vi "buffermgrModule.vi"() -> ()   [LabVIEW 2016]
uses:
  private/vis/BufferStruct.ctl
  private/vis/BUFMGR_actionStruct.ctl
panel:
  in  "error  test 2":errorcluster
  in  "autorelease":string
  in  "maxmem":u64
  in  "error  test":errorcluster
  in  "commandStruct":T1
  in  "send":bool
  in  "local cmds":string="SHUTDOWN"
  out "ConfigFile":path
  in  "log?":bool
  in  "logfile":path=path "/home/arcconfig/MOD_buffmgr.log"
  in  "configvars":string[][](table)=[["BUFF", "minimum", "buffermgrModule.vi", "minbuf", "2", "U16"], ["BUFF", "defsize", "buffermgrModule.vi", "defsize", "1900000", "U64"], ["BUFF", "maxmem", "buffermgrModule.vi", "maxmem", "", "U64"], ["BUFF", "autorelease", "buffermgrModule.vi", "autorelease", "", "STR"], ["LOG", "log", "buffermgrModule.vi", "log?", "no", "BOOL"], ["LOG", "file", "buffermgrModule.vi", "logfile", "", "PATH"]]
  out "error out":errorcluster
  in  "error in":errorcluster
  in  "module name":string="BUFMGR"
  out "automatic buff err":errorcluster
  in  "defsize":u64=19000000 caption="default buffer size"
  in  "minbuf":u16=2 caption="minimum number of free buffres to keep"
  out "stop":bool
  out "Buffers":T2[](array[typedef])
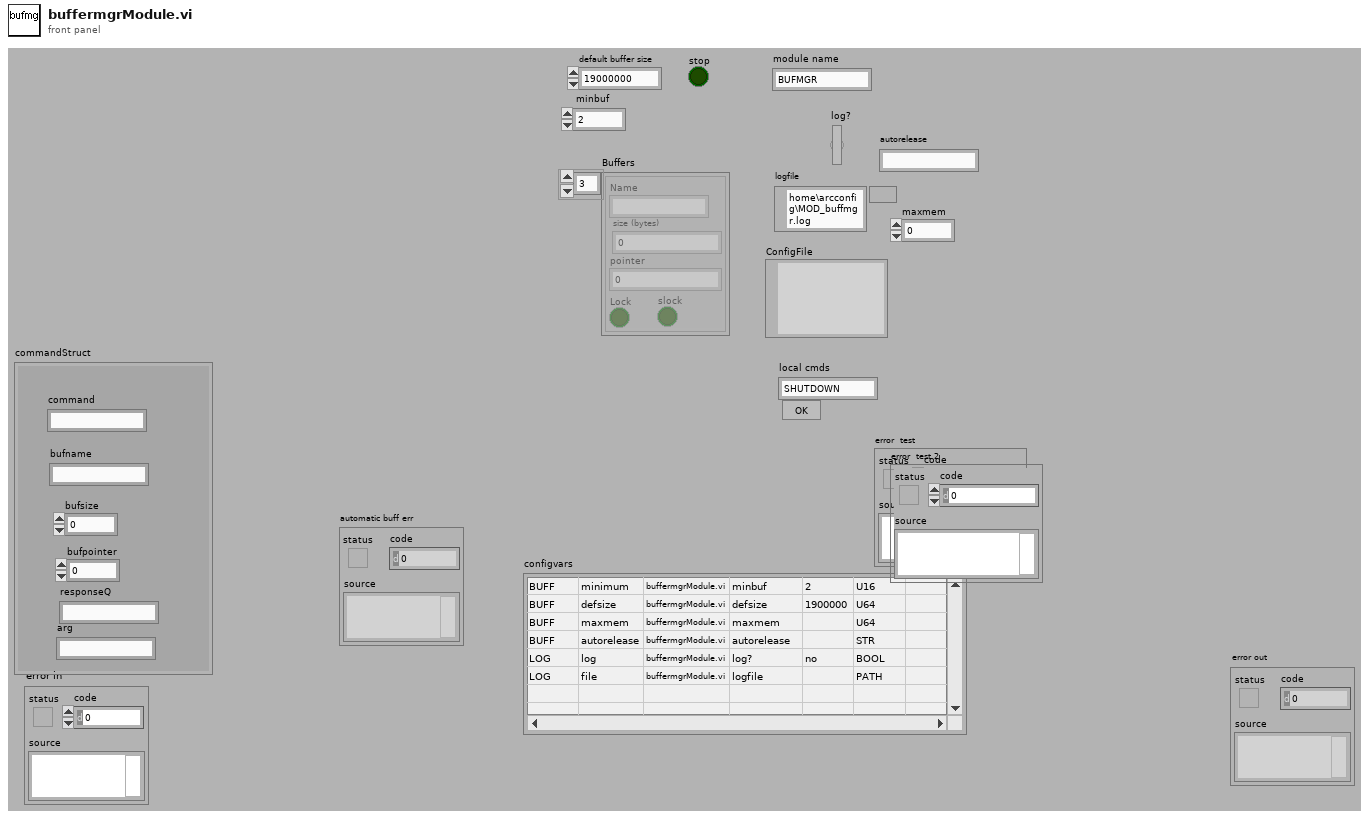
[diagram p1: front panel]
types:
  T1 = cluster{"command":string, "bufname":string, "bufsize":u64, "bufpointer":u64, "responseQ":string, "arg":string}
  T2 = typedef "BufferStruct.ctl" = cluster{"Name":string, "size (bytes)":u64, "pointer":u64, "Lock":bool, "slock":bool}
  T3 = typedef "BUFMGR_actionStruct.ctl" = enum16{"get", "release", "get & lock", "unlock", "release all", "find", "release smaller than", "release bigger than", "release different than", "release equal to", "release unlocked", "info", "get & doublelock", "release secured", "double unlock"}
  T4 = cluster{"pointer":u64, "size":u64, "progress":u32, "status":string}
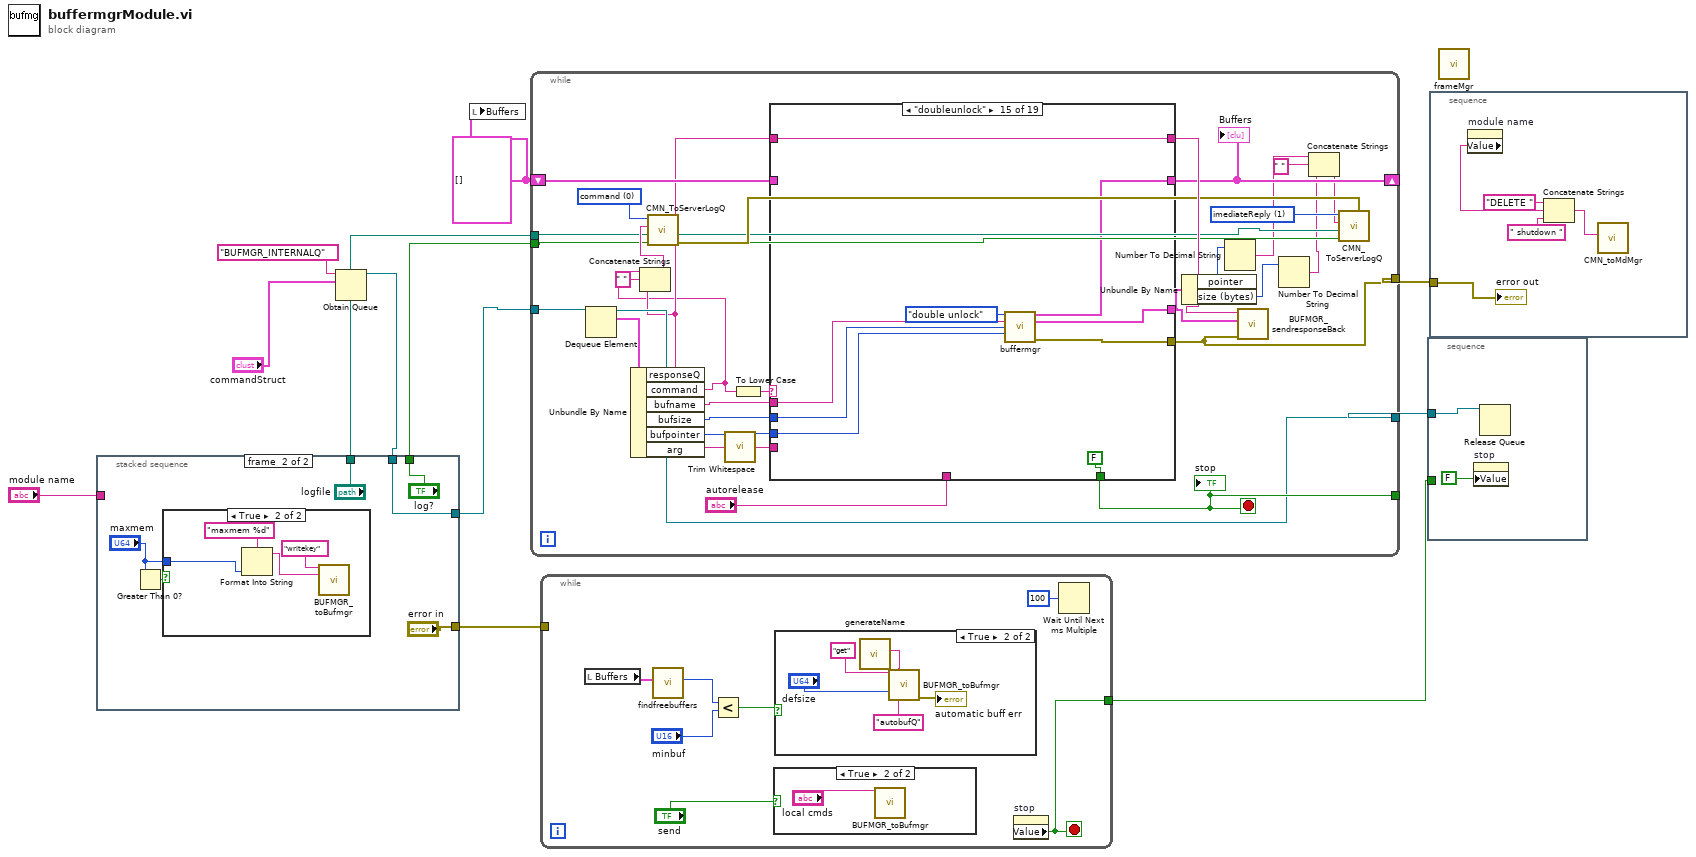
[diagram p0: block diagram]
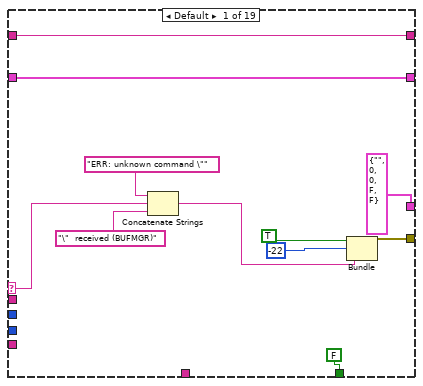
[diagram p2: hidden frame]
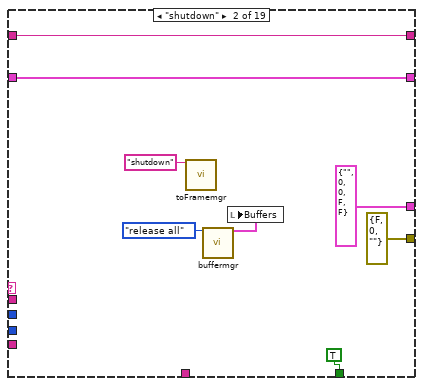
[diagram p3: hidden frame]
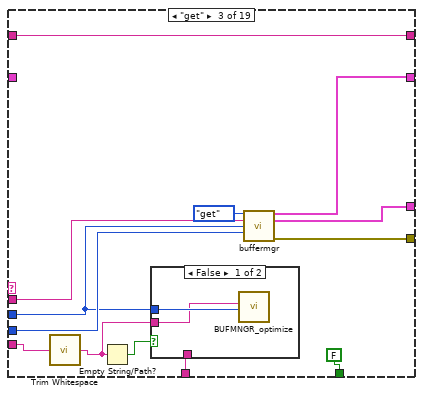
[diagram p4: hidden frame]
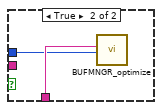
[diagram p5: hidden frame]
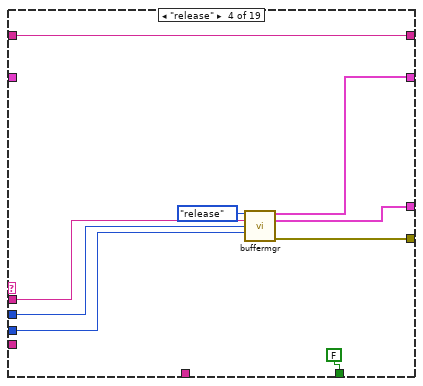
[diagram p6: hidden frame]
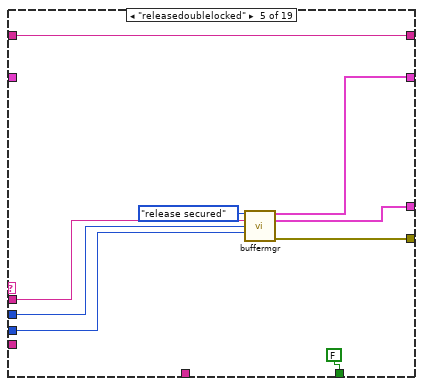
[diagram p7: hidden frame]
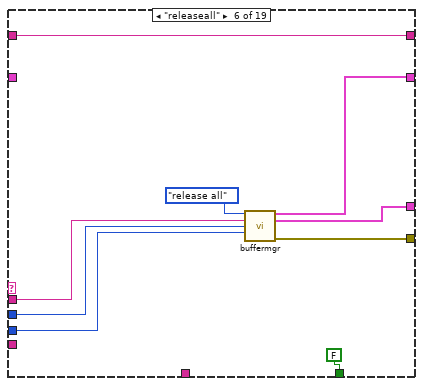
[diagram p8: hidden frame]
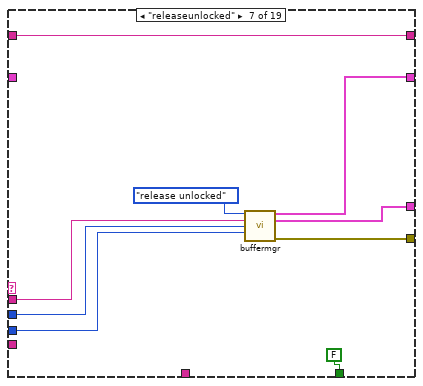
[diagram p9: hidden frame]
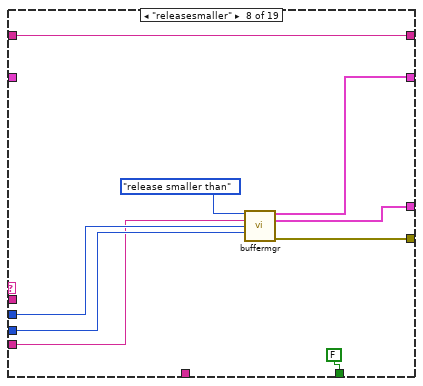
[diagram p10: hidden frame]
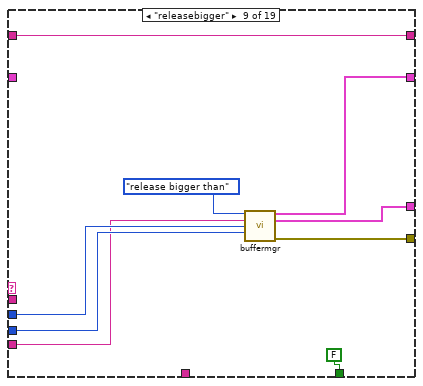
[diagram p11: hidden frame]
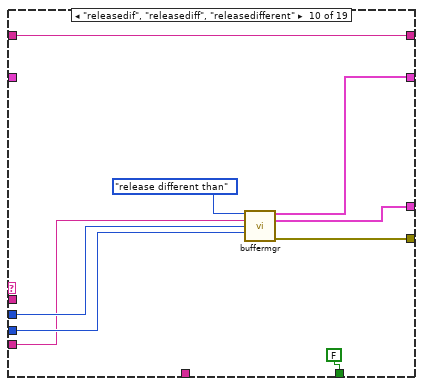
[diagram p12: hidden frame]
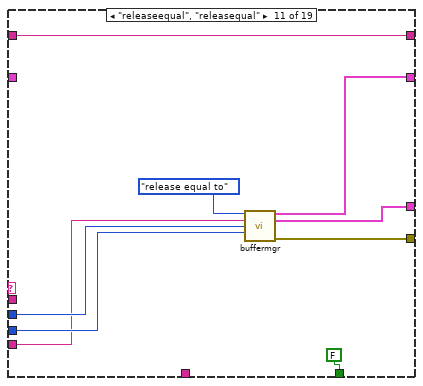
[diagram p13: hidden frame]
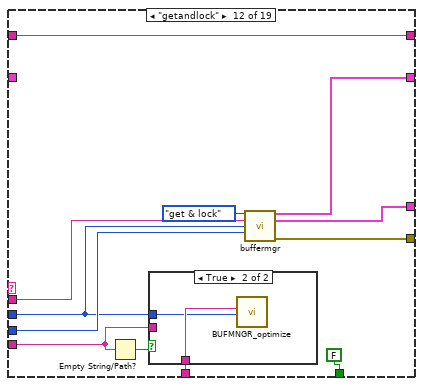
[diagram p14: hidden frame]
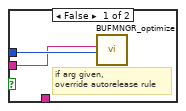
[diagram p15: hidden frame]
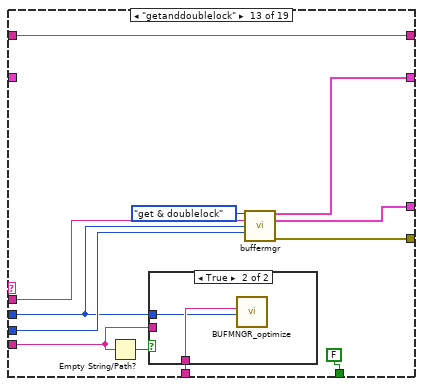
[diagram p16: hidden frame]
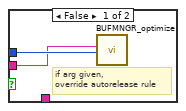
[diagram p17: hidden frame]
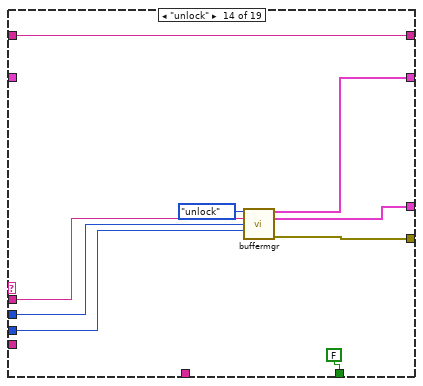
[diagram p18: hidden frame]
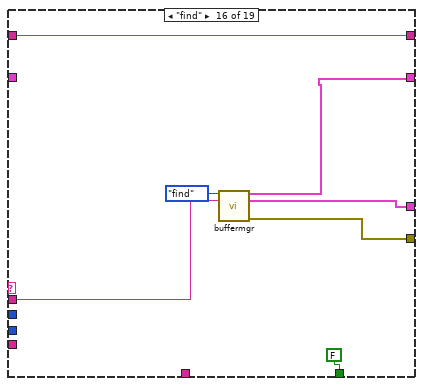
[diagram p19: hidden frame]
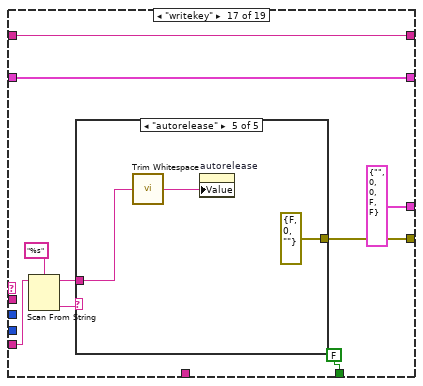
[diagram p20: hidden frame]
diagram:
  w1 = T2[] [] ("output buffers")
  n1 = Obtain Queue(name (unnamed)="BUFMGR_INTERNALQ", element data type="commandStruct") -> (queue out=w3:refnum<queue>)  [unwired: 3 in, 2 out]
  n2 = stacked-sequence {
    tunnel: [_ "error in"] -> w11
    tunnel: "module name" -> [w13 _]
    tunnel: [_ "log?"] -> w8
    tunnel: [_ "logfile"] -> w7
    tunnel: w3 -> [_ w17]
    tunnel: [_ w17] -> w2
    frame #0 {
      n3 = Current VI's Path() -> (path=w15:path)
      n4 = call "CMN_Non-standard-testpath.vi"("ModuleName"=w13, "caller Path"=w15) -> ("ConfigFile"=w14:path)  [unwired: 1 in, 8 out]
      "ConfigFile" <- w14
      n5 = call "CMN_ConfigVals.vi"("ConfigVariables"="configvars", "configuration file path"=w14) -> ()  [unwired: 2 in, 8 out]
    }
    frame #1 {
      n6 = Greater Than 0?(x="maxmem") -> (x > 0?=w19:bool)
      n7 = case shown="True" w19 {
        tunnel: "maxmem" -> [_ w25]
        frame False {
        }
        frame True {
          n8 = Format Into String(format string="maxmem %d", w25) -> (resulting string=w24:string)  [unwired: 2 in, 1 out]
          n9 = call "BUFMGR_toBufmgr.vi"("command"="writekey", "arg"=w24) -> ()  [unwired: 6 in, 8 out]
        }
      }
    }
  }
  n10 = local write "Buffers"(w1) -> ()
  n11 = while {
    tunnel: [w49] -> w10
    tunnel: [w53] -> _
    shift-left: w1 -> [w51]
    shift-right: [w50] -> _
    tunnel: w8 -> [w40]
    tunnel: w7 -> [w41]
    tunnel: [w33] -> w6
    tunnel: w2 -> [w32]
    stop <- w53 stop-if-true
    w45 = u16 1 items=["command", "imediateReply", "Callback Reply", "Information"] ("type")
    w48 = u16 0 items=["command", "imediateReply", "Callback Reply", "Information"] ("type")
    n12 = Dequeue Element(queue=w32) -> (queue out=w33:refnum<queue>, element=w34:T1)  [unwired: 1 in, 3 out]
    n13 = Unbundle By Name(w34) -> ("responseQ"=w31:string, "command"=w30:string, "bufname"=w57:string, "bufsize"=w56:u64, "bufpointer"=w55:u64, "arg"=w52:string)
    n14 = Concatenate Strings(w30, " " ("string"), w31) -> (w46:string)
    n15 = call "CMN_ToServerLogQ.vi"("Log"=w40, "file"=w41, "string"=w46, "type"=w48) -> ("error out"=w42:errorcluster)  [unwired: 2 in, 4 out]
    n16 = call <vilib>:"Trim Whitespace.vi"("string"=w52) -> ("trimmed string"=w28:string)  [unwired: 1 in]
    n17 = To Lower Case(string=w30) -> (all lower case string=w43:string)
    n18 = case shown="\"doubleunlock\"" w43 {
      selector: w43 -> [w59 _ _ _ _ _ _ _ _ _ _ _ _ _ _ _ _ _ _]
      tunnel: [FALSE TRUE FALSE FALSE FALSE FALSE FALSE FALSE FALSE FALSE FALSE FALSE FALSE FALSE FALSE FALSE FALSE FALSE FALSE] -> w53
      tunnel: w57 -> [_ _ w89 w102 w111 w120 w129 _ _ _ _ w177 w193 w206 w215 w222 _ _ _]
      tunnel: w56 -> [_ _ w80 w101 w110 w119 w128 w138 w147 w156 w165 w168 w184 w205 w214 _ _ _ _]
      tunnel: w55 -> [_ _ w88 w100 w109 w118 w127 w137 w146 w155 w164 w176 w192 w204 w213 _ _ _ _]
      tunnel: [w61 errorcluster {"status"=FALSE, "code"=0, "source"=""} ("error out") w87 w99 w108 w117 w126 w136 w145 w154 w163 w175 w191 w203 w212 w221 w225 w254 w317] -> w49
      tunnel: [T2 {"Name"="", "size (bytes)"=0, "pointer"=0, "Lock"=FALSE, "slock"=FALSE} ("output buffer") T2 {"Name"="", "size (bytes)"=0, "pointer"=0, "Lock"=FALSE, "slock"=FALSE} ("output buffer") w86 w98 w107 w116 w125 w135 w144 w153 w162 w174 w190 w202 w211 w218 T2 {"Name"="", "size (bytes)"=0, "pointer"=0, "Lock"=FALSE, "slock"=FALSE} ("output buffer") T2 {"Name"="", "size (bytes)"=0, "pointer"=0, "Lock"=FALSE, "slock"=FALSE} ("output buffer") T2 {"Name"="", "size (bytes)"=0, "pointer"=0, "Lock"=FALSE, "slock"=FALSE} ("output buffer")] -> w27
      tunnel: w31 -> [w67 w73 w84 w96 w105 w114 w123 w133 w142 w151 w160 w172 w188 w200 w209 w219 w230 w259 w322]
      tunnel: [w67 w73 w84 w96 w105 w114 w123 w133 w142 w151 w160 w172 w188 w200 w209 w219 w230 w259 w322] -> w54
      tunnel: [w66 w74 w83 w95 w104 w113 w122 w132 w141 w150 w159 w171 w187 w199 w208 w220 w231 w260 w323] -> w50
      tunnel: w51 -> [w66 w74 _ _ _ _ _ _ _ _ _ _ _ _ _ _ w231 w260 w323]
      tunnel: w28 -> [_ _ w79 _ _ _ _ w130 w139 w148 w157 w166 w182 _ _ _ w224 w252 w315]
      tunnel: "autorelease" -> [_ _ w81 _ _ _ _ _ _ _ _ w169 w185 _ _ _ _ _ _]
      frame Default {
        n19 = Concatenate Strings("ERR: unknown command \"", w59, "\"  received (BUFMGR)" ("source")) -> (w60:string)
        n20 = Bundle("status"=TRUE, "code"=-22, w60) -> (w61:cluster{"status":bool, "code":i32, string})  [unwired: 1 out]
      }
      frame "shutdown" {
        n21 = call "toFramemgr.vi"("command"="shutdown") -> ()  [unwired: 8 in, 7 out]
        n22 = call "buffermgr.vi"("Action"=BUFMGR_actionStruct."release all") -> ("output buffers"=w71:T2[])  [unwired: 4 in, 10 out]
        n23 = local write "Buffers"(w71) -> ()
      }
      frame "get" {
        n24 = call <vilib>:"Trim Whitespace.vi"("string"=w79) -> ("trimmed string"=w77:string)  [unwired: 1 in]
        n25 = Empty String/Path?(string/path=w77) -> (empty?=w78:bool)
        n26 = case shown="False" w78 {
          tunnel: w81 -> [_ w93]
          tunnel: w80 -> [w91 w92]
          tunnel: w77 -> [w90 _]
          frame False {
            n27 = call "BUFMNGR_optimize.vi"("size"=w91, "optimize"=w90) -> ()  [unwired: 10 out]
          }
          frame True {
            n28 = call "BUFMNGR_optimize.vi"("size"=w92, "optimize"=w93) -> ()  [unwired: 10 out]
          }
        }
        n29 = call "buffermgr.vi"("Action"=BUFMGR_actionStruct."get", "buffer name"=w89, "buffer size"=w80, "buffer pointer"=w88) -> ("output buffers"=w83:T2[], "output buffer"=w86:T2, "error out"=w87:errorcluster)  [unwired: 1 in, 8 out]
      }
      frame "release" {
        n30 = call "buffermgr.vi"("Action"=BUFMGR_actionStruct."release", "buffer name"=w102, "buffer size"=w101, "buffer pointer"=w100) -> ("output buffers"=w95:T2[], "output buffer"=w98:T2, "error out"=w99:errorcluster)  [unwired: 1 in, 8 out]
      }
      frame "releasedoublelocked" {
        n31 = call "buffermgr.vi"("Action"=BUFMGR_actionStruct."release secured", "buffer name"=w111, "buffer size"=w110, "buffer pointer"=w109) -> ("output buffers"=w104:T2[], "output buffer"=w107:T2, "error out"=w108:errorcluster)  [unwired: 1 in, 8 out]
      }
      frame "releaseall" {
        n32 = call "buffermgr.vi"("Action"=BUFMGR_actionStruct."release all", "buffer name"=w120, "buffer size"=w119, "buffer pointer"=w118) -> ("output buffers"=w113:T2[], "output buffer"=w116:T2, "error out"=w117:errorcluster)  [unwired: 1 in, 8 out]
      }
      frame "releaseunlocked" {
        n33 = call "buffermgr.vi"("Action"=BUFMGR_actionStruct."release unlocked", "buffer name"=w129, "buffer size"=w128, "buffer pointer"=w127) -> ("output buffers"=w122:T2[], "output buffer"=w125:T2, "error out"=w126:errorcluster)  [unwired: 1 in, 8 out]
      }
      frame "releasesmaller" {
        n34 = call "buffermgr.vi"("Action"=BUFMGR_actionStruct."release smaller than", "buffer name"=w130, "buffer size"=w138, "buffer pointer"=w137) -> ("output buffers"=w132:T2[], "output buffer"=w135:T2, "error out"=w136:errorcluster)  [unwired: 1 in, 8 out]
      }
      frame "releasebigger" {
        n35 = call "buffermgr.vi"("Action"=BUFMGR_actionStruct."release bigger than", "buffer name"=w139, "buffer size"=w147, "buffer pointer"=w146) -> ("output buffers"=w141:T2[], "output buffer"=w144:T2, "error out"=w145:errorcluster)  [unwired: 1 in, 8 out]
      }
      frame "releasedif", "releasediff", "releasedifferent" {
        n36 = call "buffermgr.vi"("Action"=BUFMGR_actionStruct."release different than", "buffer name"=w148, "buffer size"=w156, "buffer pointer"=w155) -> ("output buffers"=w150:T2[], "output buffer"=w153:T2, "error out"=w154:errorcluster)  [unwired: 1 in, 8 out]
      }
      frame "releaseequal", "releasequal" {
        n37 = call "buffermgr.vi"("Action"=BUFMGR_actionStruct."release equal to", "buffer name"=w157, "buffer size"=w165, "buffer pointer"=w164) -> ("output buffers"=w159:T2[], "output buffer"=w162:T2, "error out"=w163:errorcluster)  [unwired: 1 in, 8 out]
      }
      frame "getandlock" {
        n38 = Empty String/Path?(string/path=w166) -> (empty?=w167:bool)
        n39 = case shown="True" w167 {
          tunnel: w169 -> [_ w181]
          tunnel: w168 -> [w179 w180]
          tunnel: w166 -> [w178 _]
          frame False {
            # "if arg given,\noverride autorelease rule"
            n40 = call "BUFMNGR_optimize.vi"("size"=w179, "optimize"=w178) -> ()  [unwired: 10 out]
          }
          frame True {
            n41 = call "BUFMNGR_optimize.vi"("size"=w180, "optimize"=w181) -> ()  [unwired: 10 out]
          }
        }
        n42 = call "buffermgr.vi"("Action"=BUFMGR_actionStruct."get & lock", "buffer name"=w177, "buffer size"=w168, "buffer pointer"=w176) -> ("output buffers"=w171:T2[], "output buffer"=w174:T2, "error out"=w175:errorcluster)  [unwired: 1 in, 8 out]
      }
      frame "getanddoublelock" {
        n43 = Empty String/Path?(string/path=w182) -> (empty?=w183:bool)
        n44 = case shown="True" w183 {
          tunnel: w185 -> [_ w197]
          tunnel: w184 -> [w195 w196]
          tunnel: w182 -> [w194 _]
          frame False {
            # "if arg given,\noverride autorelease rule"
            n45 = call "BUFMNGR_optimize.vi"("size"=w195, "optimize"=w194) -> ()  [unwired: 10 out]
          }
          frame True {
            n46 = call "BUFMNGR_optimize.vi"("size"=w196, "optimize"=w197) -> ()  [unwired: 10 out]
          }
        }
        n47 = call "buffermgr.vi"("Action"=BUFMGR_actionStruct."get & doublelock", "buffer name"=w193, "buffer size"=w184, "buffer pointer"=w192) -> ("output buffers"=w187:T2[], "output buffer"=w190:T2, "error out"=w191:errorcluster)  [unwired: 1 in, 8 out]
      }
      frame "unlock" {
        n48 = call "buffermgr.vi"("Action"=BUFMGR_actionStruct."unlock", "buffer name"=w206, "buffer size"=w205, "buffer pointer"=w204) -> ("output buffers"=w199:T2[], "output buffer"=w202:T2, "error out"=w203:errorcluster)  [unwired: 1 in, 8 out]
      }
      frame "doubleunlock" {
        n49 = call "buffermgr.vi"("Action"=BUFMGR_actionStruct."double unlock", "buffer name"=w215, "buffer size"=w214, "buffer pointer"=w213) -> ("output buffers"=w208:T2[], "output buffer"=w211:T2, "error out"=w212:errorcluster)  [unwired: 1 in, 8 out]
      }
      frame "find" {
        n50 = call "buffermgr.vi"("Action"=BUFMGR_actionStruct."find", "buffer name"=w222) -> ("output buffers"=w220:T2[], "output buffer"=w218:T2, "error out"=w221:errorcluster)  [unwired: 3 in, 8 out]
      }
      frame "writekey" {
        n51 = Scan From String(format string="%s" ("Format String"), input string=w224) -> (remaining string=w226:string, output 1=w228:string)  [unwired: 2 in, 3 out]
        n52 = case shown="\"autorelease\"" w228 {
          tunnel: w226 -> [_ w235 w238 w246 w249]
          tunnel: [errorcluster {"status"=TRUE, "code"=-22, "source"="BUFMGR"} ("error out") errorcluster {"status"=FALSE, "code"=0, "source"=""} ("error out") errorcluster {"status"=FALSE, "code"=0, "source"=""} ("error out") w241 errorcluster {"status"=FALSE, "code"=0, "source"=""} ("error out")] -> w225
          frame Default {
          }
          frame "freebufs" {
            n53 = Decimal String To Number(string=w235) -> (number=w234:i32)  [unwired: 3 out]
            n54 = property on="minbuf" class="DigNum (strict)"("Value"=w234) -> ()  [unwired: 2 in, 2 out]
          }
          frame "defbufsize" {
            n55 = Decimal String To Number(string=w238) -> (number=w236:i32)  [unwired: 3 out]
            n56 = property on="defsize" class="DigNum (strict)"("Value"=w236) -> ()  [unwired: 2 in, 2 out]
          }
          frame "maxmem" {
            n57 = Scan From String(format string="%d", input string=w246, default 1=u64 0 ("default value 1")) -> (output 1=w240:u64)  [unwired: 2 in, 3 out]
            n58 = local write "maxmem"(w240) -> ()
            n59 = call "BUFMGR_set_maxmem.vi"("megs in"=w240) -> ("error out"=w243:errorcluster)  [unwired: 1 in, 13 out]
            n60 = Unbundle By Name(w243) -> ("source"=w245:string)
            n61 = Select(t=w245, s=w243, f="DONE") -> (s? t:f=w242:string)
            n62 = Bundle By Name(cluster=w243, "source"=w242) -> (w241:errorcluster)
          }
          frame "autorelease" {
            n63 = call <vilib>:"Trim Whitespace.vi"("string"=w249) -> ("trimmed string"=w248:string)  [unwired: 1 in]
            n64 = property on="autorelease" class="Str"("Value"=w248) -> ()  [unwired: 2 in, 2 out]
          }
        }
      }
      frame "info" {
        n65 = Scan From String(format string="%s" ("Format String"), input string=w252) -> (remaining string=w255:string, output 1=w257:string)  [unwired: 2 in, 3 out]
        n66 = case shown="\"defbufsize\"" w257 {
          selector: w257 -> [w263 _ _ _ _ _ _ _ _]
          tunnel: w255 -> [_ _ _ _ _ _ _ _ _]
          tunnel: [w261 w265 w276 w283 w287 w291 w297 w303 w308] -> w254
          tunnel: "error  test" -> [_ w266 w277 w284 w288 w292 w298 w304 w311]
          frame Default {
            n67 = call "CMN_BadParamMsg.vi"("valid params"=string[] ["minfreebufs", "totmem", "defbufsize", "maxmem", "buflist", "logfile", "configfile", "logging"], "parameter"=w263) -> ("error out"=w261:errorcluster)  [unwired: 2 in, 7 out]
          }
          frame "freebufs", "minbufs", "minfreebufs" {
            n68 = property on="minbuf" class="DigNum (strict)"() -> ("Value"=w264:u16)  [unwired: 2 in, 2 out]
            n69 = Format Into String(w264) -> (resulting string=w267:string)  [unwired: 3 in, 1 out]
            n70 = Bundle By Name(cluster=w266, "status"=FALSE, "code"=0, "source"=w267) -> (w265:errorcluster)
          }
          frame "maxmem" {
            n71 = call "BUFMGR_get_maxmem.vi"() -> ("return"=w275:u64)  [unwired: 1 in, 14 out]
            n72 = Format Into String(format string="%ld [Mb]", w275) -> (resulting string=w273:string)  [unwired: 2 in, 1 out]
            n73 = Less Or Equal To 0?(x=w275) -> (x <= 0?=w274:bool)
            n74 = Select(t="NONE", s=w274, f=w273) -> (s? t:f=w271:string)
            n75 = Bundle By Name(cluster=w277, "status"=FALSE, "code"=0, "source"=w271) -> (w276:errorcluster)
          }
          frame "totmem" {
            n76 = call "BUFMGR_get_totmem.vi"() -> ("return"=w282:u64)  [unwired: 1 in, 14 out]
            n77 = Format Into String(format string="%ld [Mb]", w282) -> (resulting string=w280:string)  [unwired: 2 in, 1 out]
            n78 = Bundle By Name(cluster=w284, "status"=FALSE, "code"=0, "source"=w280) -> (w283:errorcluster)
          }
          frame "buffers", "buffs", "buflist", "bufs" {
            n79 = call "BUFMGR_bufs2str.vi"() -> ("buffers"=w289:string)  [unwired: 11 out]
            n80 = Bundle By Name(cluster=w288, "source"=w289) -> (w287:errorcluster)
          }
          frame "logfile" {
            n81 = property on="logfile" class="Path"() -> ("Value"=w290:path)  [unwired: 2 in, 2 out]
            n82 = Format Into String(w290) -> (resulting string=w293:string)  [unwired: 3 in, 1 out]
            n83 = Bundle By Name(cluster=w292, "status"=FALSE, "code"=0, "source"=w293) -> (w291:errorcluster)
          }
          frame "configfile" {
            n84 = property on="ConfigFile" class="Path"() -> ("Value"=w296:path)  [unwired: 2 in, 2 out]
            n85 = Format Into String(w296) -> (resulting string=w299:string)  [unwired: 3 in, 1 out]
            n86 = Bundle By Name(cluster=w298, "status"=FALSE, "code"=0, "source"=w299) -> (w297:errorcluster)
          }
          frame "logging" {
            n87 = property on="log?" class="Bool (strict)"() -> ("Value"=w302:bool)  [unwired: 2 in, 2 out]
            n88 = Format Into String(w302) -> (resulting string=w305:string)  [unwired: 3 in, 1 out]
            n89 = Bundle By Name(cluster=w304, "status"=FALSE, "code"=0, "source"=w305) -> (w303:errorcluster)
          }
          frame "defbufsize" {
            n90 = property on="defsize" class="DigNum (strict)"() -> ("Value"=w310:u64)  [unwired: 2 in, 2 out]
            n91 = Format Into String(w310) -> (resulting string=w309:string)  [unwired: 3 in, 1 out]
            n92 = Bundle By Name(cluster=w311, "status"=FALSE, "code"=0, "source"=w309) -> (w308:errorcluster)
          }
        }
      }
      frame "frame", "frameinfo" {
        n93 = Scan From String(format string="%s" ("Format String"), input string=w315) -> (remaining string=w318:string, output 1=w320:string)  [unwired: 2 in, 3 out]
        n94 = case shown="\"index\"" w320 {
          selector: w320 -> [w326 _ _ _]
          tunnel: w318 -> [_ w336 _ _]
          tunnel: [w324 w331 w343 w353] -> w317
          tunnel: "error  test 2" -> [_ w330 w342 w352]
          frame Default {
            n95 = call "CMN_BadParamMsg.vi"("valid params"=string[] ["minfreebufs", "totmem", "defbufsize", "maxmem", "buflist", "logfile", "configfile", "logging"], "parameter"=w326) -> ("error out"=w324:errorcluster)  [unwired: 2 in, 7 out]
          }
          frame "index" {
            n96 = call "toFramemgr.vi"("command"="get", "arg"=w336, "responseQ"="bufmgr2framemgrq") -> ("buffer"=w335:T4)  [unwired: 6 in, 6 out]
            n97 = Unbundle By Name(w335) -> ("pointer"=w334:u64, "progress"=w333:u32)
            n98 = Format Into String(format string="0x%x (%d)", w334, w333) -> (resulting string=w328:string)  [unwired: 2 in, 1 out]
            n99 = Bundle By Name(cluster=w330, "status"=FALSE, "source"=w328, "code"=0) -> (w331:errorcluster)
          }
          frame "numframes", "size" {
            n100 = call "toFramemgr.vi"("command"="info", "responseQ"="bufmgr2framemgrq") -> ("buffer"=w346:T4)  [unwired: 7 in, 6 out]
            n101 = Unbundle By Name(w346) -> ("size"=w345:u64)
            n102 = Format Into String(format string="%d", w345) -> (resulting string=w340:string)  [unwired: 2 in, 1 out]
            n103 = Bundle By Name(cluster=w342, "status"=FALSE, "source"=w340, "code"=0) -> (w343:errorcluster)
          }
          frame "deleteall" {
            n104 = call "toFramemgr.vi"("command"="deleteall", "responseQ"="bufmgr2framemgrq") -> ()  [unwired: 7 in, 7 out]
            n105 = Bundle By Name(cluster=w352, "status"=FALSE, "source"="DONE", "code"=0) -> (w353:errorcluster)
          }
        }
      }
    }
    "stop" <- w53
    "Buffers" <- w50
    n106 = Unbundle By Name(w27) -> ("pointer"=w44:u64, "size (bytes)"=w39:u64)
    n107 = Number To Decimal String(number=w44) -> (decimal integer string=w38:string)  [unwired: 1 out]
    n108 = call "BUFMGR_sendresponseBack.vi"("error in (no error)"=w49, "buffer"=w27, "Qname"=w54) -> ()  [unwired: 8 out]
    n109 = Number To Decimal String(number=w39) -> (decimal integer string=w36:string)  [unwired: 1 out]
    n110 = Concatenate Strings(w38, " " ("string"), w36) -> (w35:string)
    n111 = call "CMN_ToServerLogQ.vi"("error in (no error)"=w42, "Log"=w40, "file"=w41, "string"=w35, "type"=w45) -> ()  [unwired: 1 in, 5 out]
  }
  n112 = while {
    tunnel: w11 -> [_]
    tunnel: [w357] -> w12
    stop <- w357 stop-if-true
    n113 = local read "Buffers"() -> (w361:T2[])
    n114 = call "findfreebuffers.vi"("Buffers"=w361) -> ("unlock buffers"=w360:i32)  [unwired: 10 out]
    n115 = Less?(x=w360, y="minbuf") -> (x < y?=w358:bool)
    n116 = case shown="True" "send" {
      frame False {
      }
      frame True {
        n117 = call "BUFMGR_toBufmgr.vi"("command"="local cmds") -> ()  [unwired: 7 in, 8 out]
      }
    }
    n118 = case shown="True" w358 {
      frame False {
      }
      frame True {
        n119 = call "generateName.vi"() -> ("buffername"=w366:string)  [unwired: 10 out]
        n120 = call "BUFMGR_toBufmgr.vi"("command"="get", "bufname"=w366, "bufsize"="defsize", "responseQ"="autobufQ") -> ("error out"=→"automatic buff err":errorcluster)  [unwired: 4 in, 7 out]
      }
    }
    n121 = property on="stop" class="Bool (strict)"() -> ("Value"=w357:bool)  [unwired: 2 in, 2 out]
    n122 = Wait Until Next ms Multiple(millisecond multiple=u32 100) -> ()  [unwired: 1 out]
  }
  n123 = stacked-sequence {
    tunnel: w12 -> [_]
    tunnel: w6 -> [w369]
    frame #0 {
      n124 = property on="stop" class="Bool (strict)"("Value"=FALSE ("stop")) -> ()  [unwired: 2 in, 2 out]
      n125 = Release Queue(queue=w369) -> ()  [unwired: 1 in, 4 out]
    }
  }
  n126 = stacked-sequence {
    tunnel: w10 -> [w375]
    frame #0 {
      n127 = property on="module name" class="Str"() -> ("Value"=w371:string)  [unwired: 2 in, 2 out]
      n128 = Concatenate Strings("DELETE " ("string"), w371, " shutdown ") -> (w372:string)
      n129 = call "CMN_toMdMgr.vi"("command"=w372) -> ()  [unwired: 10 out]
      "error out" <- w375
    }
  }
  n130 = call "frameMgr.vi"() -> ()  [unwired: 1 out]
